vi "GEOM_NOAOCalculateHeadersS.vi"(0 "datacols":u16, 1 "type":u16(ring) items=["LL", "LR", "UL", "UR"], 2 "amp ID":string, 3 "Corrected ROI":T1={"xstart"=1, "ystart"=1, "xsize"=1, "ysize"=1}, 4 "det ID":string, 5 "datarows":u16, 6 "ME Headers":string[][](table)=[["AMPSEC", "[1:1,1:1]", "amplifier section", "STRING"], ["CCDSEC", "[1:1,1:1]", "ccd section", "STRING"], ["CCDSIZE", "[1:1,1:1]", "ccd size", "STRING"], ["TRIMSEC", "[1:1,1:1]", "trim section", "STRING"], ["DATASEC", "[1:1,1:1]", "data section", "STRING"], ["BIASSEC", "", "bias section", "STRING"], ["DETSEC", "[0:0,0:0]", "detector section", "STRING"]], 7 "trims":u16, 9 "overscan":u16, 10 "Req  ROI":T1={"xstart"=1, "ystart"=1, "xsize"=1, "ysize"=1}, 11 "bias skip begining":u16, 12 "xstart":i32, 13 "ystart":i32, 14 "Binning":cluster{"x":u32, "y":u32}={"x"=1, "y"=1} {"y" min=1; "x" min=1}, 15 "ytrims":i32) -> (8 "S headers out":string[][](table)=[["ASEC", "", "amplifier section", "STRING"], ["BSEC", "", "bias section", "STRING"], ["CSEC", "", "section read in FULL ccd for DSEC", "STRING"], ["DSEC", "", "image area in raw frame", "STRING"], ["TSEC", "", "trim section", "STRING"]])   [LabVIEW 2016]
panel:
  in  "keyword table":string[][](table)=[["ASEC", "", "amplifier section", "STRING"], ["BSEC", "", "bias section", "STRING"], ["CSEC", "", "section in full ccd for DSEC", "STRING"], ["DSEC", "", "image section in raw frame", "STRING"], ["TSEC", "", "trim section", "STRING"]]
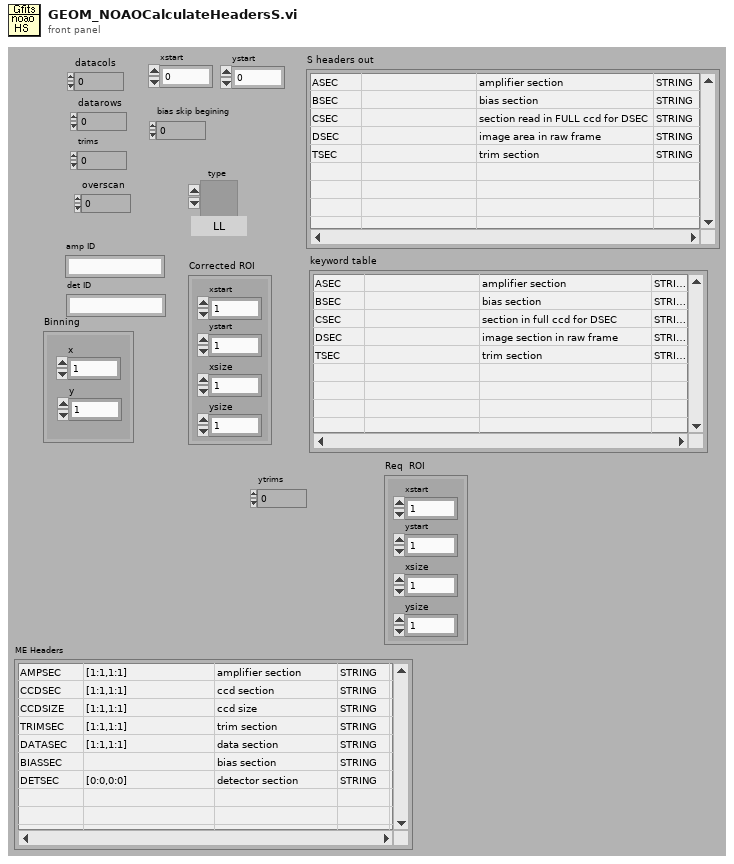
[diagram p1: front panel]
types:
  T1 = cluster{"xstart":u32, "ystart":u32, "xsize":u32, "ysize":u32}
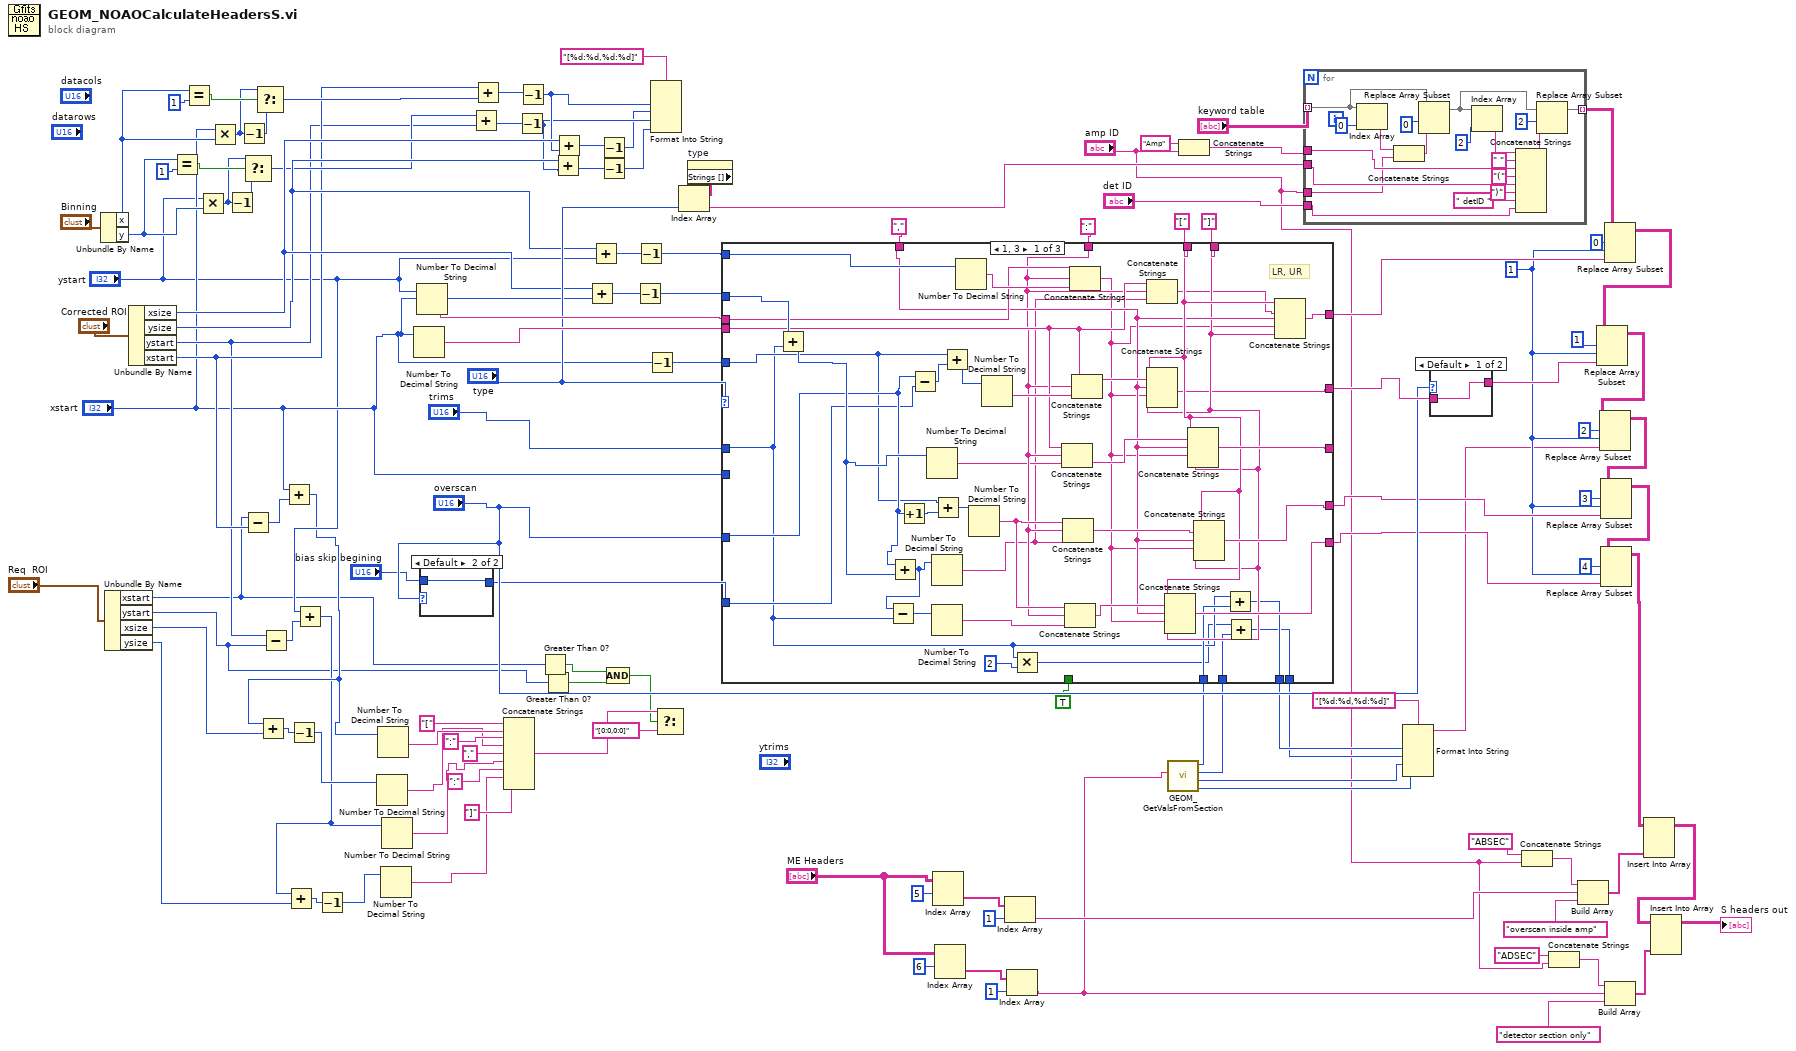
[diagram p0: block diagram]
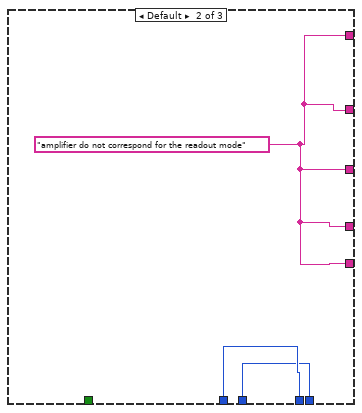
[diagram p2: hidden frame]
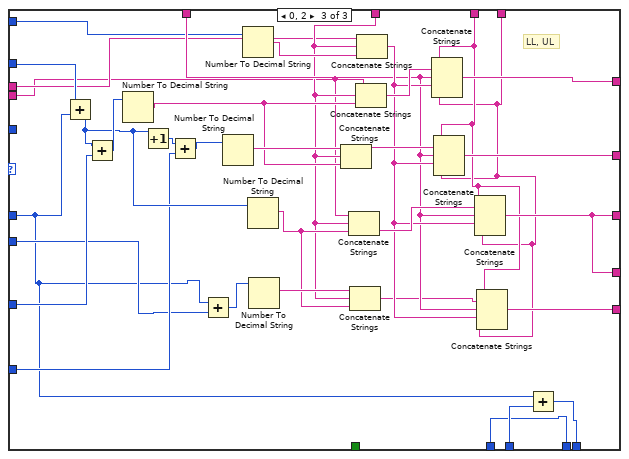
[diagram p3: hidden frame]
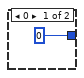
[diagram p4: hidden frame]
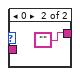
[diagram p5: hidden frame]
diagram:
  w62 = 1 ("disabled index (col)")
  n1 = Unbundle By Name("Binning") -> ("x"=w77:u32, "y"=w70:u32)
  n2 = Unbundle By Name("Req  ROI") -> ("xstart"=w40:u32, "ystart"=w35:u32, "xsize"=w50:u32, "ysize"=w44:u32)
  n3 = Unbundle By Name("Corrected ROI") -> ("xsize"=w86:u32, "ysize"=w84:u32, "ystart"=w63:u32, "xstart"=w64:u32)
  n4 = Equal?(x=w70, y=u32 1) -> (x = y?=w74:bool)
  n5 = Equal?(x=w77, y=u32 1) -> (x = y?=w80:bool)
  n6 = Multiply(x="ystart", y=w70) -> (x*y=w73:u32)
  n7 = Multiply(x="xstart", y=w77) -> (x*y=w79:u32)
  n8 = Decrement(x=w73) -> (x-1=w72:u32)
  n9 = Decrement(x=w79) -> (x-1=w78:u32)
  n10 = Select(t=w73, s=w74, f=w72) -> (s? t:f=w71:u32)
  n11 = Subtract(x=w40, y=w64) -> (x-y=w58:u32)
  n12 = Select(t=w79, s=w80, f=w78) -> (s? t:f=w76:u32)
  n13 = Subtract(x=w63, y=w35) -> (x-y=w57:u32)
  n14 = Add(x="xstart", y=w58) -> (x+y=w51:u32)
  n15 = Add(x=w51, y=w50) -> (x+y=w49:u32)
  n16 = Decrement(x=w49) -> (x-1=w42:u32)
  n17 = Add(x="ystart", y=w57) -> (x+y=w41:u32)
  n18 = Add(x=w41, y=w44) -> (x+y=w45:u32)
  n19 = Decrement(x=w45) -> (x-1=w43:u32)
  n20 = Number To Decimal String(number=w42) -> (decimal integer string=w48:string)  [unwired: 1 out]
  n21 = Number To Decimal String(number=w51) -> (decimal integer string=w60:string)  [unwired: 1 out]
  n22 = Number To Decimal String(number=w43) -> (decimal integer string=w46:string)  [unwired: 1 out]
  n23 = Number To Decimal String(number=w41) -> (decimal integer string=w47:string)  [unwired: 1 out]
  n24 = Number To Decimal String(number="xstart") -> (decimal integer string=w118:string)  [unwired: 1 out]
  n25 = Number To Decimal String(number="ystart") -> (decimal integer string=w119:string)  [unwired: 1 out]
  n26 = case shown="Default" "overscan" {
    tunnel: [0 w126] -> w121
    tunnel: "bias skip begining" -> [_ w126]
    frame 0 {
    }
    frame Default {
    }
  }
  n27 = Add(x=w71, y=w63) -> (x+y=w90:u32)
  n28 = Add(x=w64, y=w76) -> (x+y=w89:u32)
  n29 = Concatenate Strings("[" ("string"), w60, ":" ("string"), w48, "," ("string"), w47, ":" ("string"), w46, "]" ("string")) -> (w38:string)
  n30 = Decrement(x=w90) -> (x-1=w69:u32)
  n31 = Decrement(x=w89) -> (x-1=w85:u32)
  n32 = Greater Than 0?(x=w40) -> (x > 0?=w37:bool)
  n33 = Greater Than 0?(x=w35) -> (x > 0?=w34:bool)
  n34 = Add(x=w84, y=w69) -> (x+y=w88:u32)
  n35 = Add(x=w86, y=w85) -> (x+y=w87:u32)
  n36 = Add(x=w86, y="xstart") -> (x+y=w112:u32)
  n37 = Add(x=w84, y="ystart") -> (x+y=w113:u32)
  n38 = Decrement(x=w87) -> (x-1=w68:u32)
  n39 = Decrement(x=w88) -> (x-1=w67:u32)
  n40 = Compound Arithmetic op=AND(w37, w34) -> (w36:bool)
  n41 = Decrement(x=w112) -> (x-1=w110:u32)
  n42 = Decrement(x=w113) -> (x-1=w111:u32)
  n43 = Decrement(x="xstart") -> (x-1=w109:i32)
  n44 = Format Into String(format string="[%d:%d,%d:%d]", w85, w68, w69, w67) -> ()  [unwired: 2 in, 2 out]
  n45 = Select(t=w38, s=w36, f="[0:0,0:0]") -> ()  [unwired: 1 out]
  n46 = property on="type" class="Ring (strict)"() -> ("Strings []"=w93:string[])  [unwired: 2 in, 2 out]
  n47 = Index Array(array=w93, index="type") -> (element=w18:string)
  n48 = Index Array(array="ME Headers", index (row)=5) -> (element=w32:string[])  [unwired: 1 in]
  n49 = Index Array(array="ME Headers", index (row)=6) -> (element=w29:string[])  [unwired: 1 in]
  n50 = Index Array(array=w32, index=1) -> (element=w15:string)
  n51 = Index Array(array=w29, index=1) -> (element=w13:string)
  n52 = call "GEOM_GetValsFromSection.vi"("section"=w13) -> ("yend"=w10:i32, "ystart"=w11:i32, "xend"=w8:i32, "xstart"=w9:i32)  [unwired: 7 out]
  n53 = case shown="1, 3" "type" {
    tunnel: w111 -> [w156 _ w181]
    tunnel: w110 -> [w157 _ w180]
    tunnel: "trims" -> [w128 _ w175]
    tunnel: "overscan" -> [w155 _ w198]
    tunnel: "," ("dim separator") -> [w143 _ w192]
    tunnel: [w140 w171 w203] -> w108
    tunnel: [w141 w171 w199] -> w124
    tunnel: [w153 w171 w196] -> _
    tunnel: [w152 w171 w196] -> w101
    tunnel: [w151 w171 w188] -> w98
    tunnel: "[" -> [w144 _ w187]
    tunnel: "]" -> [w142 _ w186]
    tunnel: ":" ("pixel separator") -> [w138 _ w185]
    tunnel: w121 -> [w154 _ w182]
    tunnel: TRUE -> [_ _ _]
    tunnel: w119 -> [w150 _ w179]
    tunnel: w118 -> [w139 _ w178]
    tunnel: w109 -> [w146 _ _]
    tunnel: "xstart" -> [_ _ w176]
    tunnel: w9 -> [w133 w170 w173]
    tunnel: w8 -> [w132 w169 w174]
    tunnel: [w131 w170 w173] -> w7
    tunnel: [w130 w169 w172] -> w6
    frame 1, 3 {
      # "LR, UR"
      n54 = Add(x=w157, y=w128) -> (x+y=w158:u32)
      n55 = Add(x=w155, y=w158) -> (x+y=w162:u32)
      n56 = Subtract(x=w162, y=w128) -> (x-y=w163:u32)
      n57 = Increment(x=w155) -> (x+1=w147:u16)
      n58 = Subtract(x=w155, y=w154) -> (x-y=w149:i32)
      n59 = Number To Decimal String(number=w158) -> (decimal integer string=w135:string)  [unwired: 1 out]
      n60 = Number To Decimal String(number=w162) -> (decimal integer string=w134:string)  [unwired: 1 out]
      n61 = Number To Decimal String(number=w163) -> (decimal integer string=w161:string)  [unwired: 1 out]
      n62 = Add(x=w146, y=w147) -> (x+y=w145:i32)
      n63 = Add(x=w146, y=w149) -> (x+y=w148:i32)
      n64 = Number To Decimal String(number=w156) -> (decimal integer string=w168:string)  [unwired: 1 out]
      n65 = Number To Decimal String(number=w145) -> (decimal integer string=w160:string)  [unwired: 1 out]
      n66 = Number To Decimal String(number=w148) -> (decimal integer string=w164:string)  [unwired: 1 out]
      n67 = Multiply(x=w128, y=u16 2) -> (x*y=w127:u16)
      n68 = Concatenate Strings(w139, w138, w135) -> (w166:string)
      n69 = Concatenate Strings(w160, w138, w134) -> (w165:string)
      n70 = Concatenate Strings(w160, w138, w161) -> (w159:string)
      n71 = Concatenate Strings(w150, w138, w168) -> (w136:string)
      n72 = Concatenate Strings(w139, w138, w164) -> (w167:string)
      n73 = Concatenate Strings(w139, w138, w134) -> (w137:string)
      n74 = Concatenate Strings(w144, w167, w143, w136, w142) -> (w141:string)
      n75 = Concatenate Strings(w144, w159, w143, w136, w142) -> (w151:string)
      n76 = Concatenate Strings(w144, w166, w143, w136, w142) -> (w153:string)
      n77 = Concatenate Strings(w144, w165, w143, w136, w142) -> (w152:string)
      n78 = Add(x=w128, y=w133) -> (x+y=w131:i32)
      n79 = Add(x=w127, y=w132) -> (x+y=w130:i32)
      n80 = Concatenate Strings(w144, w137, w143, w136, w142) -> (w140:string)
    }
    frame Default {
      w171 = "amplifier do not correspond for the readout mode"
    }
    frame 0, 2 {
      # "LL, UL"
      n81 = Add(x=w180, y=w175) -> (x+y=w194:u32)
      n82 = Add(x=w194, y=w198) -> (x+y=w195:u32)
      n83 = Number To Decimal String(number=w195) -> (decimal integer string=w201:string)  [unwired: 1 out]
      n84 = Increment(x=w194) -> (x+1=w184:u32)
      n85 = Add(x=w184, y=w182) -> (x+y=w183:u32)
      n86 = Add(x=w175, y=w176) -> (x+y=w177:i32)
      n87 = Number To Decimal String(number=w183) -> (decimal integer string=w202:string)  [unwired: 1 out]
      n88 = Number To Decimal String(number=w181) -> (decimal integer string=w205:string)  [unwired: 1 out]
      n89 = Number To Decimal String(number=w194) -> (decimal integer string=w190:string)  [unwired: 1 out]
      n90 = Number To Decimal String(number=w177) -> (decimal integer string=w191:string)  [unwired: 1 out]
      n91 = Concatenate Strings(w202, w185, w201) -> (w200:string)
      n92 = Concatenate Strings(w178, w185, w190) -> (w197:string)
      n93 = Concatenate Strings(w191, w185, w190) -> (w189:string)
      n94 = Concatenate Strings(w178, w185, w201) -> (w204:string)
      n95 = Concatenate Strings(w179, w185, w205) -> (w193:string)
      n96 = Concatenate Strings(w187, w204, w192, w193, w186) -> (w203:string)
      n97 = Concatenate Strings(w187, w200, w192, w193, w186) -> (w199:string)
      n98 = Concatenate Strings(w187, w197, w192, w193, w186) -> (w196:string)
      n99 = Concatenate Strings(w187, w189, w192, w193, w186) -> (w188:string)
      n100 = Add(x=w175, y=w174) -> (x+y=w172:i32)
    }
  }
  n101 = Concatenate Strings("Amp" ("string"), "amp ID") -> (w3:string)
  n102 = for {
    tunnel: "keyword table" -> [w222] mode=indexing
    tunnel: w3 -> [w214]
    tunnel: [w209] -> w94 mode=indexing
    tunnel: w18 -> [w211]
    tunnel: "det ID" -> [w207]
    tunnel: "amp ID" -> [w206]
    n103 = Index Array(array=w222, index=0) -> (element=w221:string)
    n104 = Concatenate Strings(w221, w206) -> (w220:string)
    n105 = Replace Array Subset(array=w222, new element=w220, index=0) -> (w218:string[])
    n106 = Index Array(array=w218, index=2) -> (element=w216:string)
    n107 = Concatenate Strings(w216, " " ("string"), w214, "(" ("string"), w211, ")" ("string"), " detID " ("string"), w207) -> (w210:string)
    n108 = Replace Array Subset(array=w218, new element=w210, index=2) -> (w209:string[])
  }
  n109 = Format Into String(format string="[%d:%d,%d:%d]", w7, w6, w11, w10) -> (resulting string=w5:string)  [unwired: 2 in, 1 out]
  n110 = case shown="Default" "overscan" {
    tunnel: w124 -> [w225 _]
    tunnel: [w225 ""] -> w106
    frame Default {
    }
    frame 0 {
    }
  }
  n111 = Concatenate Strings("ABSEC" ("string"), "amp ID") -> (w25:string)
  n112 = Concatenate Strings("ADSEC" ("string"), "amp ID") -> (w20:string)
  n113 = Build Array(w25, w15, "overscan inside amp" ("element")) -> (w23:string[])
  n114 = Replace Array Subset(array=w94, new element=w108, index (row)=0, index (col)=w62) -> (w96:string[][])
  n115 = Replace Array Subset(array=w96, new element=w106, index (row)=1 ("index (col)"), index (col)=w62) -> (w104:string[][])
  n116 = Replace Array Subset(array=w104, new element=w5, index (row)=2 ("disabled index (row)"), index (col)=w62) -> (w103:string[][])
  n117 = Replace Array Subset(array=w103, new element=w101, index (row)=3, index (col)=w62) -> (w99:string[][])
  n118 = Replace Array Subset(array=w99, new element=w98, index (row)=4, index (col)=w62) -> (w2:string[][])
  n119 = Build Array(w20, w13, "detector section only" ("element")) -> (w17:string[])
  n120 = Insert Into Array(array=w2, new element=w23) -> (w22:string[][])  [unwired: 2 in]
  n121 = Insert Into Array(array=w22, new element=w17) -> (→"S headers out":string[][])  [unwired: 2 in]
